vi "Open_Instr.vi"(8 "error in (no error)":errorcluster caption="entrée d'erreur (pas d'erreur)", 11 "Class Multimeter (Default) en entrée":refnum<class "Class Instrument Printer.lvclass">) -> (0 "error out":errorcluster caption="sortie d'erreur", 3 "Class Multimeter (Default) en sortie":refnum<class "Class Instrument Printer.lvclass">)   [LabVIEW 2020, in "Library Instrument & Equipement.lvlib" / "Library Instruments.lvlib" / "Class Instrument Printer.lvclass"]
doc: "Opens and acquires an instrument"
uses:
  Class Instrument Printer.lvclass
  Class Instrument Printer.lvclass/Class Instrument Printer.ctl
  Instrument (Default)/Class Instrument (Default).lvclass
  Printer/Printer (Default)/Class Printer (Default).lvclass
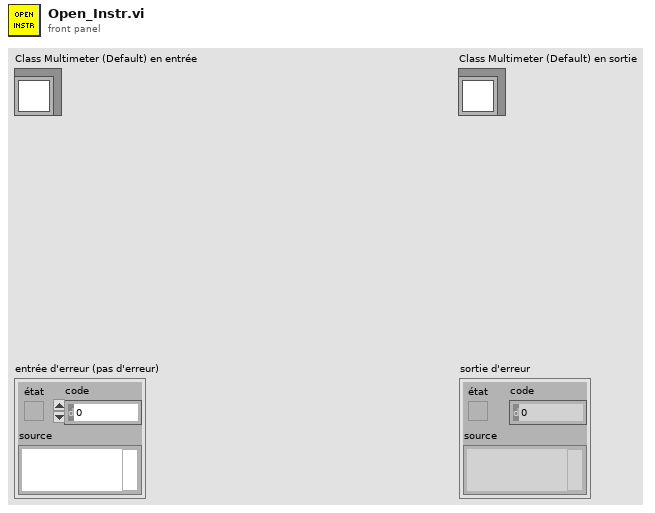
[diagram p1: front panel]
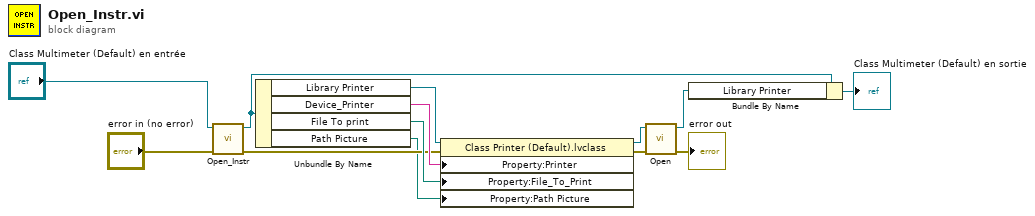
[diagram p0: block diagram]
diagram:
  n1 = call-parent "Open_Instr.vi"("error in (no error)"="error in (no error)", "Class Multimeter (Default) en entrée"="Class Multimeter (Default) en entrée") -> ("error out"=w8:errorcluster, "Class Multimeter (Default) en sortie"=w3:refnum<class "Class Instrument Printer.lvclass">)  [unwired: 8 in]
  n2 = Unbundle By Name(w3) -> ("Library Printer"=w11:refnum<class "Class Printer (Default).lvclass">, "Device_Printer"=w10:string, "File To print"=w9:path, "Path Picture"=w1:path)
  n3 = property class="Class Printer (Default).lvclass"(reference=w11, error in=w8, "Property:Printer"=w10, "Property:File_To_Print"=w9, "Property:Path Picture"=w1) -> (reference out=w6:refnum<class "Class Printer (Default).lvclass">, error out=w7:errorcluster)
  n4 = call-dynamic "Open.vi"("error in (no error)"=w7, "Class Printer (Default) en entrée"=w6) -> ("error out"=→"error out":errorcluster, "Class Printer (Default) en sortie"=w4:refnum<class "Class Printer (Default).lvclass">)  [unwired: 8 in]
  n5 = Bundle By Name(cluster=w3, "Library Printer"=w4) -> (→"Class Multimeter (Default) en sortie":refnum<class "Class Instrument Printer.lvclass">)
